vi "OpenDSForReading.vi"(3 "DS Server\nIP Address":string="dstp://localshost/wave") -> (0 "error out":errorcluster, 1 "DataSocket Refnum":refnum<k13>)   [LabVIEW 2011]
panel:
  in  "mode":T1(ring)=enum."ReadWrite"
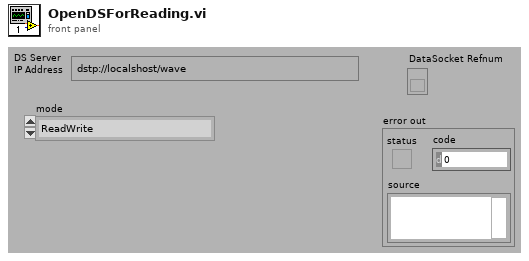
[diagram p1: front panel]
types:
  T1 = enum16{"Read", "Write", "ReadWrite", "BufferedRead", "BufferedReadWrite"}
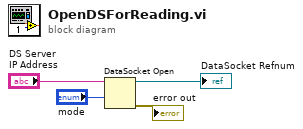
[diagram p0: block diagram]
diagram:
  n1 = DataSocket Open(10:"mode", 11:"DS Server\nIP Address") -> (0:→"error out":errorcluster, 3:→"DataSocket Refnum":refnum<k13>)  [unwired: 1 in, 1 out]
